vi "Term_Project_FM.vi"() -> ()   [LabVIEW 2012]
doc: "This VI illustrates how to perform simultaneous sound IO, i.e., how to continuously play the sound acquired from a microphone. It requires the use of a microphone attached to the sound card. You can specify the IDs of the input and output devices, the frequency to sample at, and the buffer size for both devices. Higher frequencies have better quality, but demand more resources and are limited by the capabilities of your sound card. A large number of samples decreases the risk of glitches, but increases the delay between acquisition and playback."
uses:
  <vilib>/sound2/lvsound2.llb/Sound Data Format.ctl
  <vilib>/sound2/lvsound2.llb/Sampling Mode.ctl
  <vilib>/sound2/lvsound2.llb/Sound Output Write (DBL Single).vi
  <instrlib>/niUSRP/niUSRP Fetch Rx Data (CDB Cluster).vi
  <instrlib>/niUSRP/niUSRP Write Tx Data (CDB Cluster).vi
  <vilib>/sound2/lvsound2.llb/Sound Input Read (DBL).vi
  <vilib>/addons/Modulation/niAMT.lvlib
panel:
  in  "carrier frequency":u16(ring) items=["500 MHz", "300 MHz", "200 MHz"]
  in  "Amplifying Index":dbl(slide)=1.0 scale=0.0..100.0
  in  "FM deviation (Hz)":dbl(slide)=300000.0 scale=20000.0..30000.0
  in  "Press":bool
  out "FM modulated waveform":cluster{"t0":dbl, "dt":dbl, "Y":cdb[]} {"Y" format="%.2f"; "dt" format="%.2f"; "t0" format="%.2f"}
  out "Demodulated Output":waveform(dbl)(graph)
  out "Stop 2":bool
  in  "Output Device ID":u32
  out "error out":errorcluster
  in  "active antenna":string="RX2"
  out "actual gain (dB)":dbl format="%#_6f"
  in  "gain (dB) (Rx)":dbl format="%#_6f"
  out "actual carrier frequency":dbl=100000.0 format="%#_6p"
  out "actual IQ rate (Rx)":dbl=100000.0 format="%#_6p"
  in  "IQ rate (Rx)":dbl=1000000.0 format="%#_6p"
  in  "device names":refnum<k15>="192.168.10.2"
  in  "active antenna (Tx)":string="TX1"
  out "actual gain (dB) (Tx)":dbl format="%#_6f"
  in  "gain (dB) (Tx)":dbl format="%#_6f"
  out "actual carrier frequency (Tx)":dbl=100000.0 format="%#_6p"
  out "actual IQ rate (Tx)":dbl=100000.0 format="%#_6p"
  in  "IQ rate (Tx)":dbl=200000.0 format="%#_6p"
  in  "Tx device":refnum<k15>="192.168.10.2"
  in  "carrier frequency":u16(ring) items=["500 MHz", "300 MHz", "200 MHz"]
  out "Message":waveform(dbl)[](graph)
  in  "Stop":bool
  in  "Input Device ID":u32
  # "TRANSMITTING"
  # "CONTROL"
  # "RECEIVING"
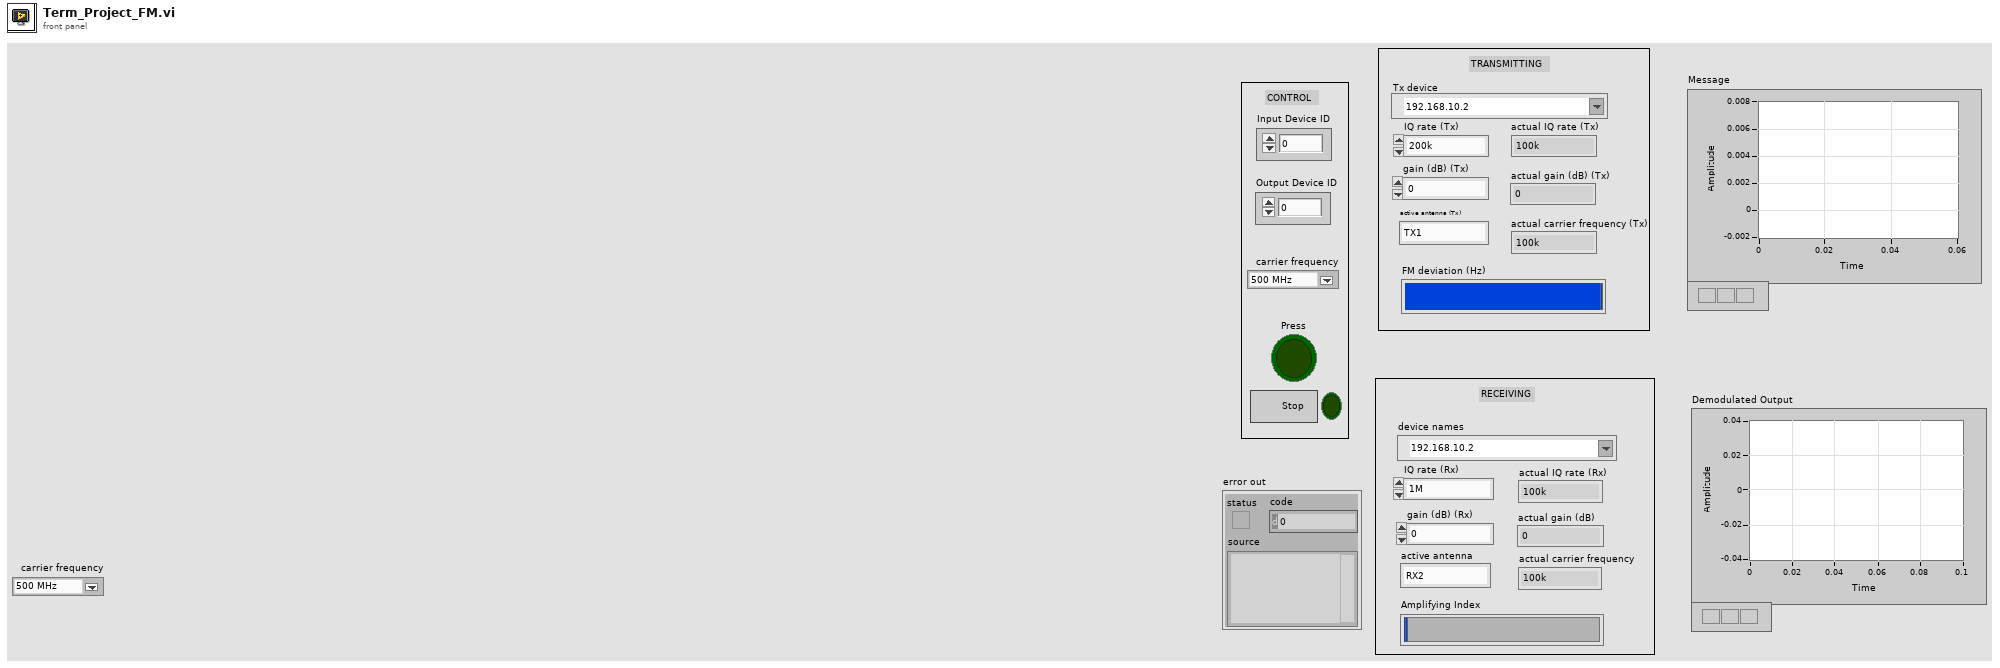
[diagram p1: front panel]
types:
  T1 = typedef "Sampling Mode.ctl" = i32
  T2 = typedef "Sound Data Format.ctl" = cluster{"sample rate (S/s)":dbl, "number of channels":i32, "bits per sample":i32}
  T3 = typedef "Sound Input Task ID.ctl" = u32
  T4 = typedef "Sound Output Task ID.ctl" = u32
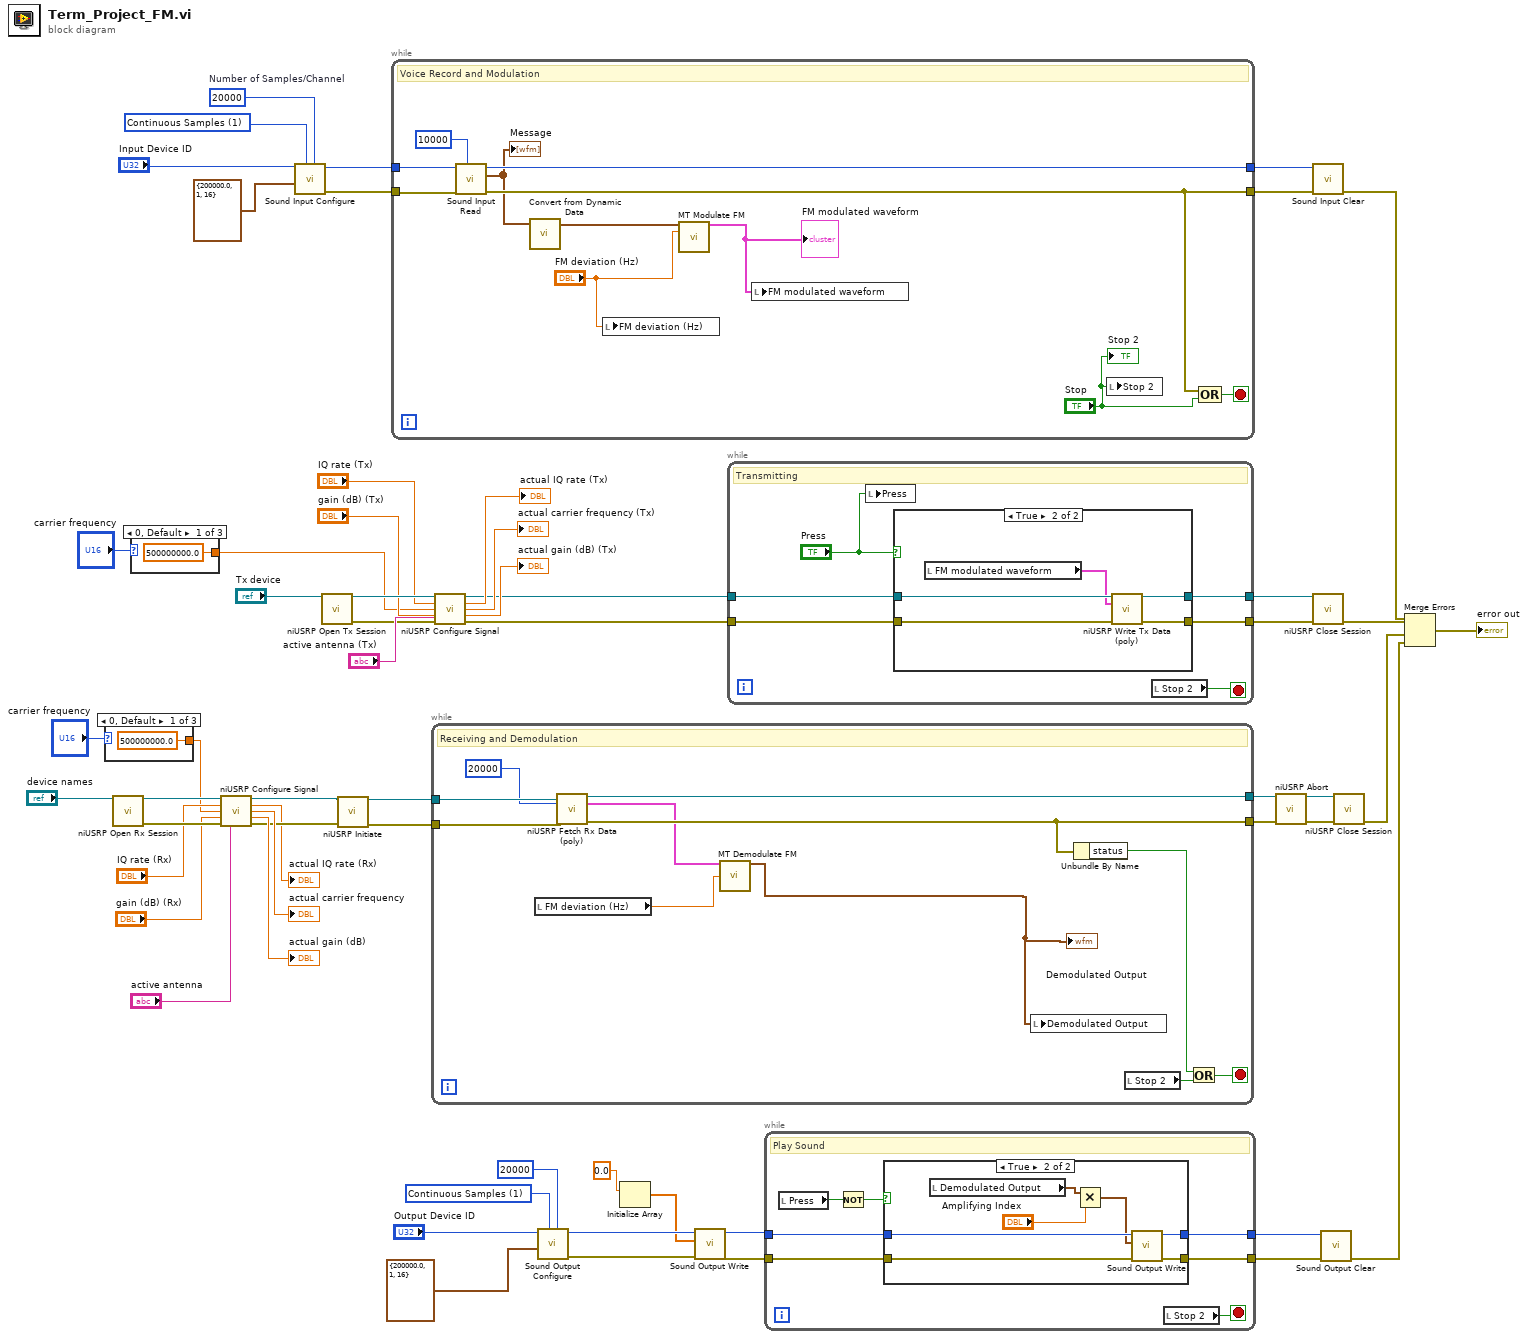
[diagram p0: block diagram]
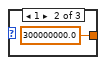
[diagram p2: hidden frame]
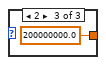
[diagram p3: hidden frame]
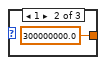
[diagram p6: hidden frame]
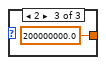
[diagram p7: hidden frame]
diagram:
  w15 = T1 1 items=["Finite Samples", "Continuous Samples"] ("sample mode")
  w51 = 20000  # Number of Samples/Channel
  w52 = T1 1 items=["Finite Samples", "Continuous Samples"] ("sample mode")
  n1 = case shown="0, Default" "carrier frequency" {
    tunnel: [500000000.0 ("sample rate (S/s)") 300000000.0 ("sample rate (S/s)") 200000000.0 ("sample rate (S/s)")] -> w1
    frame 0, Default {
    }
    frame 1 {
    }
    frame 2 {
    }
  }
  n2 = call <instrlib>:"niUSRP Open Rx Session.vi"("device names"="device names") -> ("session handle out"=w36:refnum<k15>, "error out"=w35:errorcluster)  [unwired: 13 in]
  n3 = case shown="0, Default" "carrier frequency" {
    tunnel: [500000000.0 ("sample rate (S/s)") 300000000.0 ("sample rate (S/s)") 200000000.0 ("sample rate (S/s)")] -> w7
    frame 0, Default {
    }
    frame 1 {
    }
    frame 2 {
    }
  }
  n4 = call <instrlib>:"niUSRP Configure Signal.vi"("session handle"=w36, "IQ rate"="IQ rate (Rx)", "carrier frequency"=w1, "gain"="gain (dB) (Rx)", "error in (no error)"=w35, "active antenna"="active antenna") -> ("session handle out"=w30:refnum<k15>, "coerced IQ rate"=→"actual IQ rate (Rx)":dbl, "coerced carrier frequency"=→"actual carrier frequency":dbl, "coerced gain"=→"actual gain (dB)":dbl, "error out"=w29:errorcluster)  [unwired: 5 in]
  n5 = call <vilib>:"Sound Input Configure.vi"("number of samples/ch"=w51, "sample mode"=w52, "sound format"=T2 {"sample rate (S/s)"=200000.0, "number of channels"=1, "bits per sample"=16} ("Sound Format"), "device ID"="Input Device ID") -> ("error out"=w55:errorcluster, "task ID"=w54:T3)  [unwired: 6 in]
  n6 = call <instrlib>:"niUSRP Open Tx Session.vi"("device names"="Tx device") -> ("session handle out"=w48:refnum<k15>, "error out"=w44:errorcluster)  [unwired: 13 in]
  n7 = call <instrlib>:"niUSRP Initiate.vi"("session handle"=w30, "error in (no error)"=w29) -> ("session handle out"=w27:refnum<k15>, "error out"=w26:errorcluster)  [unwired: 12 in]
  n8 = while {
    tunnel: w54 -> [w74]
    tunnel: [w76] -> w57
    tunnel: w55 -> [w73]
    tunnel: [w71] -> w59
    stop <- w75 stop-if-true
    # "Voice Record and Modulation"
    n9 = call-poly <vilib>:"Sound Input Read.vi"("number of samples/ch"=10000, "error in (no error)"=w73, "task ID"=w74) -> ("error out"=w71:errorcluster, "data"=w69:waveform(dbl)[], "task ID out"=w76:T3)  [unwired: 6 in]
    "Message" <- w69
    n10 = call "Convert from Dynamic Data"("Dynamic Data Type"=w69) -> ("Waveform"=w66:waveform(dbl))  [unwired: 3 in]
    n11 = local write "FM deviation (Hz)"("FM deviation (Hz)") -> ()
    n12 = call <vilib>:"MT Modulate FM.vi"("message signal"=w66, "FM deviation (Hz)"="FM deviation (Hz)") -> ("FM modulated waveform"=w68:cluster{"t0":dbl, "dt":dbl, "Y":cdb[]})  [unwired: 12 in, 1 out]
    "FM modulated waveform" <- w68
    n13 = local write "FM modulated waveform"(w68) -> ()
    n14 = local write "Stop 2"("Stop") -> ()
    n15 = Compound Arithmetic op=OR(w71, "Stop") -> (w75:bool)
    "Stop 2" <- "Stop"
  }
  n16 = while {
    tunnel: w27 -> [w87]
    tunnel: w26 -> [w86]
    tunnel: [w85] -> w25
    tunnel: [w82] -> w24
    stop <- w84 stop-if-true
    # "Receiving and Demodulation"
    n17 = local read "FM deviation (Hz)"() -> (w78:dbl)
    n18 = call-poly <instrlib>:"niUSRP Fetch Rx Data (poly).vi"("session handle"=w87, "number of samples"=i64 20000, "error in (no error)"=w86) -> ("session handle out"=w85:refnum<k15>, "data"=w79:cluster{"t0":dbl, "dt":dbl, "Y":cdb[]}, "error out"=w82:errorcluster)  [unwired: 9 in, 1 out]
    n19 = call <vilib>:"MT Demodulate FM.vi"("FM modulated waveform"=w79, "FM deviation (Hz)"=w78) -> ("FM demodulated waveform"=w77:waveform(dbl))  [unwired: 11 in, 2 out]
    "Demodulated Output" <- w77
    n20 = local write "Demodulated Output"(w77) -> ()
    n21 = Unbundle By Name(w82) -> ("status"=w83:bool)
    n22 = local read "Stop 2"() -> (w80:bool)
    n23 = Or(x=w83, y=w80) -> (x .or. y?=w84:bool)
  }
  n24 = call <instrlib>:"niUSRP Configure Signal.vi"("session handle"=w48, "IQ rate"="IQ rate (Tx)", "carrier frequency"=w7, "gain"="gain (dB) (Tx)", "error in (no error)"=w44, "active antenna"="active antenna (Tx)") -> ("session handle out"=w39:refnum<k15>, "coerced IQ rate"=→"actual IQ rate (Tx)":dbl, "coerced carrier frequency"=→"actual carrier frequency (Tx)":dbl, "coerced gain"=→"actual gain (dB) (Tx)":dbl, "error out"=w38:errorcluster)  [unwired: 5 in]
  n25 = call <vilib>:"Sound Output Configure.vi"("number of samples/ch"=20000, "sample mode"=w15, "sound format"=T2 {"sample rate (S/s)"=200000.0, "number of channels"=1, "bits per sample"=16} ("Sound Format"), "device ID"="Output Device ID") -> ("error out"=w18:errorcluster, "task ID"=w19:T4)  [unwired: 6 in]
  n26 = Initialize Array(0.0 ("element")) -> (w16:dbl[])  [unwired: 1 in]
  n27 = call-poly <vilib>:"Sound Output Write.vi"("error in (no error)"=w18, "data"=w16, "task ID"=w19) -> ("error out"=w3:errorcluster, "task ID out"=w4:T4)  [unwired: 7 in]
  n28 = while {
    tunnel: w39 -> [w93]
    tunnel: [w92] -> w12
    tunnel: [w91] -> w13
    tunnel: w38 -> [w90]
    stop <- w89 stop-if-true
    # "Transmitting"
    n29 = local write "Press"("Press") -> ()
    n30 = case shown="True" "Press" {
      tunnel: w93 -> [w95 w100]
      tunnel: [w95 w99] -> w92
      tunnel: [w94 w98] -> w91
      tunnel: w90 -> [w94 w97]
      frame False {
      }
      frame True {
        n31 = local read "FM modulated waveform"() -> (w96:cluster{"t0":dbl, "dt":dbl, "Y":cdb[]})
        n32 = call-poly <instrlib>:"niUSRP Write Tx Data (poly).vi"("session handle"=w100, "data"=w96, "error in (no error)"=w97) -> ("session handle out"=w99:refnum<k15>, "error out"=w98:errorcluster)  [unwired: 11 in]
      }
    }
    n33 = local read "Stop 2"() -> (w89:bool)
  }
  n34 = while {
    tunnel: [w107] -> w5
    tunnel: [w106] -> w6
    tunnel: w4 -> [w105]
    tunnel: w3 -> [w104]
    stop <- w103 stop-if-true
    # "Play Sound"
    n35 = local read "Press"() -> (w101:bool)
    n36 = Not(x=w101) -> (.not. x?=w102:bool)
    n37 = case shown="True" w102 {
      tunnel: [w109 w116] -> w107
      tunnel: [w108 w115] -> w106
      tunnel: w105 -> [w109 w114]
      tunnel: w104 -> [w108 w113]
      frame False {
      }
      frame True {
        n38 = local read "Demodulated Output"() -> (w112:waveform(dbl))
        n39 = Multiply(x=w112, y="Amplifying Index") -> (x*y=w110:waveform(dbl))
        n40 = call-poly <vilib>:"Sound Output Write.vi"("error in (no error)"=w113, "data"=w110, "task ID"=w114) -> ("error out"=w115:errorcluster, "task ID out"=w116:T4)  [unwired: 7 in]
      }
    }
    n41 = local read "Stop 2"() -> (w103:bool)
  }
  n42 = call <instrlib>:"niUSRP Abort.vi"("session handle"=w25, "error in (no error)"=w24) -> ("session handle out"=w23:refnum<k15>, "error out"=w22:errorcluster)  [unwired: 12 in]
  n43 = call <vilib>:"Sound Input Clear.vi"("error in (no error)"=w59, "task ID"=w57) -> ("error out"=w56:errorcluster)  [unwired: 9 in]
  n44 = call <instrlib>:"niUSRP Close Session.vi"("session handle"=w12, "error in (no error)"=w13) -> ("error out"=w50:errorcluster)  [unwired: 13 in]
  n45 = call <vilib>:"Sound Output Clear.vi"("error in (no error)"=w6, "task ID"=w5) -> ("error out"=w9:errorcluster)  [unwired: 9 in]
  n46 = call <instrlib>:"niUSRP Close Session.vi"("session handle"=w23, "error in (no error)"=w22) -> ("error out"=w10:errorcluster)  [unwired: 13 in]
  n47 = Merge Errors(w56, w50, w10, w9) -> (→"error out":errorcluster)
